vi "setTiming(private).vi"(8 "error in (no error)":errorcluster, 10 "Timing":T1={"Sampling"={"Fs"=1000.0, "#s"=128}, "sample mode"=10123, "FsMode"=enum."Manual", "Fs Multiplier"=1.0, "Refresh Rate (Hz)"=10.0, "Decimation.PreDSP"=1, "Decimation.PostDSP"=1, "Fs.Output"=204789.0} {"Sampling"."Fs" format="%#_13g"}, 11 "DAQmx in":refnum<class "DAQmx.lvclass">) -> (0 "error out":errorcluster, 3 "DAQmx out":refnum<class "DAQmx.lvclass">)   [LabVIEW 2019, in "DAQmx.lvclass"]
uses:
  DAQmx.lvclass
  typedefs/DAQ.Config.Timing.Sampling--Cluster.ctl
  typedefs/DAQ.Config.Timing.Fs Mode--enum.ctl
  typedefs/DAQ.Config.Timing--Cluster.ctl
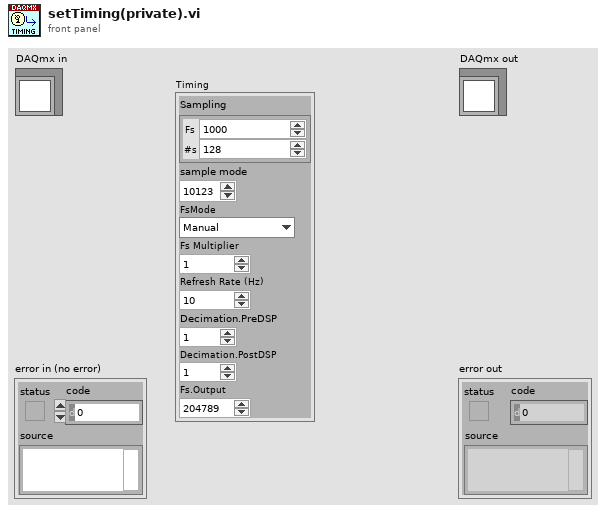
[diagram p1: front panel]
types:
  T1 = typedef "DAQmx.lvclass/DAQ.Config.Timing--Cluster.ctl" = cluster{"Sampling":T2, "sample mode":i32, "FsMode":T3, "Fs Multiplier":dbl, "Refresh Rate (Hz)":dbl, "Decimation.PreDSP":i32, "Decimation.PostDSP":i32, "Fs.Output":dbl}
  T2 = typedef "DAQmx.lvclass/DAQ.Config.Timing.Sampling--Cluster.ctl" = cluster{"Fs":dbl, "#s":i32}
  T3 = typedef "DAQmx.lvclass/DAQ.Config.Timing.Fs Mode--enum.ctl" = enum16{"Manual", "Auto Fs", "Max Fs"}
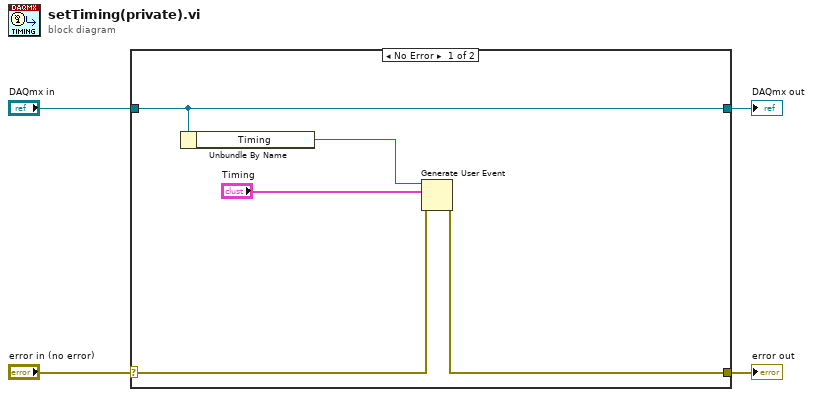
[diagram p0: block diagram]
diagram:
  n1 = case shown="No Error" "error in (no error)" {
    selector: "error in (no error)" -> [w7 w11]
    tunnel: [w6 w11] -> w3
    tunnel: [w9 w10] -> w1
    tunnel: "DAQmx in" -> [w9 w10]
    frame No Error {
      n2 = Unbundle By Name(w9) -> ("Timing"=w8:refnum<user-event>)
      n3 = Generate User Event(user event=w8, event data cluster="Timing", error in=w7) -> (error out=w6:errorcluster)  [unwired: 1 in, 1 out]
    }
    frame Error {
    }
  }
  "error out" <- w3
  "DAQmx out" <- w1
